vi "Execute Tests.vi"(7 "Suite Label":string, 8 "error in (no error)":errorcluster, 11 "Unit Tests for Runner in":refnum<class "Unit Tests for Runner.lvclass">) -> (0 "error out":errorcluster, 3 "Unit Tests for Runner out":refnum<class "Unit Tests for Runner.lvclass">)   [LabVIEW 2013, in "Unit Tests for Runner.lvclass"]
uses:
  Unit Tests for Runner.lvclass
  classes/Test Runner/Test Runner.lvclass
  classes/Assert/Assert.lvclass
  classes/Test/Test.lvclass
panel:
  out "test passed":bool
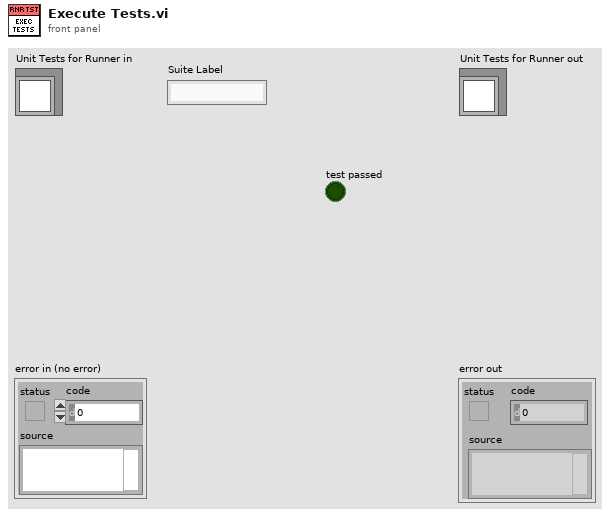
[diagram p1: front panel]
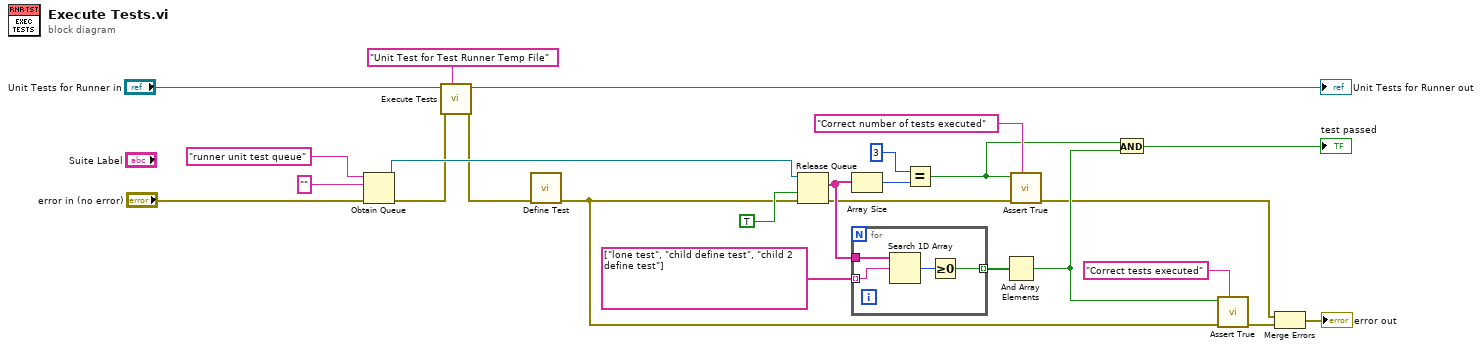
[diagram p0: block diagram]
diagram:
  n1 = Obtain Queue(name (unnamed)="runner unit test queue", element data type="", error in (no error)="error in (no error)") -> (queue out=w5:refnum<queue>, error out=w2:errorcluster)  [unwired: 2 in, 1 out]
  n2 = call-parent "Execute Tests.vi"("Suite Label"="Unit Test for Test Runner Temp File", "error in (no error)"=w2, "Test Runner in"="Unit Tests for Runner in") -> ("error out"=w1:errorcluster, "Test Runner out"=→"Unit Tests for Runner out":refnum<class "Unit Tests for Runner.lvclass">)  [unwired: 7 in]
  n3 = call "Define Test.vi"("error in (no error)"=w1) -> ("error out"=w11:errorcluster)  [unwired: 10 in]
  n4 = Release Queue(queue=w5, force destroy? (F)=TRUE, error in (no error)=w11) -> (remaining elements=w22:string[], error out=w18:errorcluster)  [unwired: 1 out]
  n5 = Array Size(array=w22) -> (size(s)=w21:i32)
  n6 = for {
    tunnel: w22 -> [w29]
    tunnel: string[] ["lone test", "child define test", "child 2 define test"] -> [w28] mode=indexing
    tunnel: [w26] -> w17 mode=indexing
    n7 = Search 1D Array(1D array=w29, element=w28) -> (index of element=w27:i32)  [unwired: 1 in]
    n8 = Greater Or Equal To 0?(x=w27) -> (x >= 0?=w26:bool)
  }
  n9 = Equal?(x=3, y=w21) -> (x = y?=w13:bool)
  n10 = And Array Elements(Boolean array=w17) -> (logical AND=w14:bool)
  n11 = call "Assert True.vi"("Label"="Correct number of tests executed", "error in (no error)"=w18, "True?"=w13) -> ("error out"=w9:errorcluster)  [unwired: 8 in]
  n12 = And(x=w13, y=w14) -> (x .and. y?=→"test passed":bool)
  n13 = call "Assert True.vi"("Label"="Correct tests executed", "error in (no error)"=w11, "True?"=w14) -> ("error out"=w15:errorcluster)  [unwired: 8 in]
  n14 = Merge Errors(w9, w15) -> (→"error out":errorcluster)
